vi "Reorder Connector Pane Object Refs.vi"(8 "Error In":errorcluster, 10 "Connector Pane Patter":u32, 11 "Connector Pane Object Refs":refnum<vi>[](array[refnum])) -> (0 "Error Out":errorcluster, 3 "Connector Pane Object Refs":refnum<vi>[][](array[refnum]))   [LabVIEW 2011, in "LVH-Toolbox.lvlib" / "LVH-Front-Panel-Clean-Up.lvlib"]
uses:
  <vilib>/LabVIEW Hacker/LVH-Toolbox/Front Panel Clean Up/LVH-Front-Panel-Clean-Up.lvlib
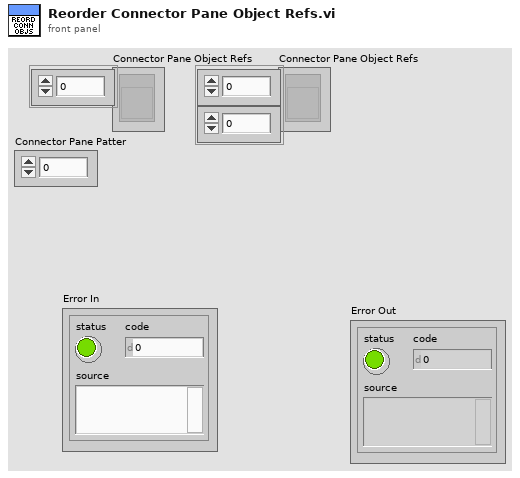
[diagram p1: front panel]
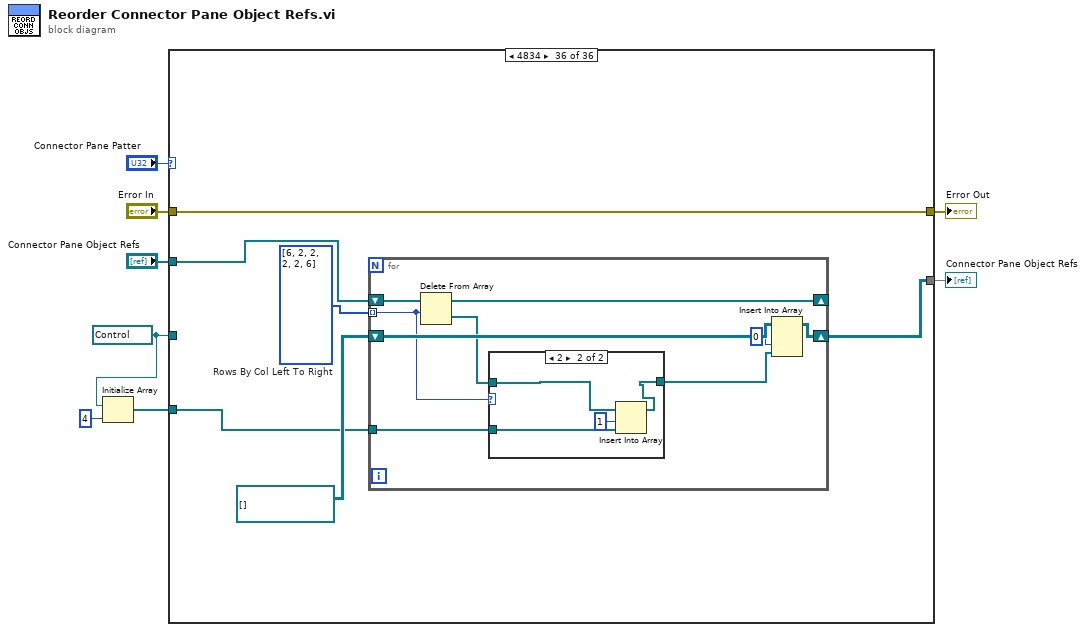
[diagram p0: block diagram]
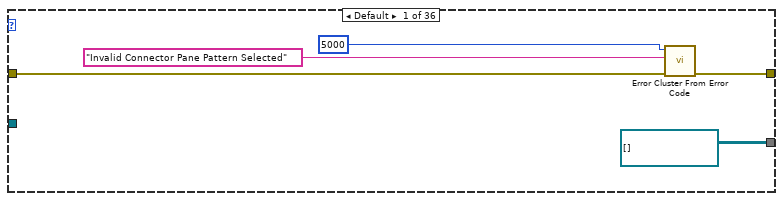
[diagram p2: hidden frame]
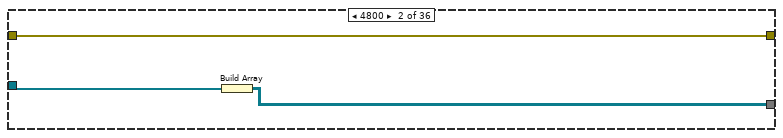
[diagram p3: hidden frame]
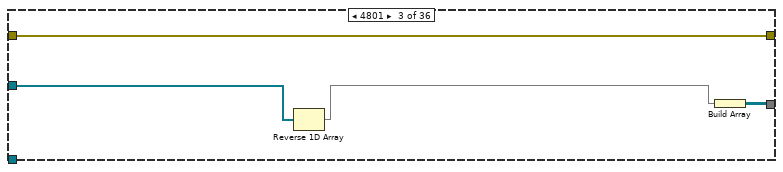
[diagram p4: hidden frame]
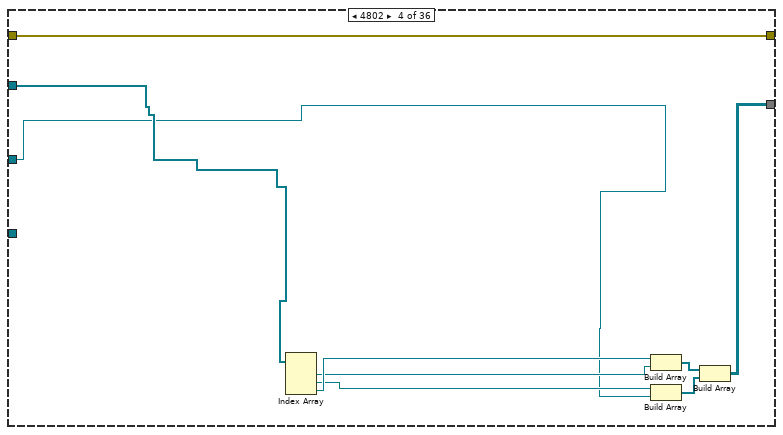
[diagram p5: hidden frame]
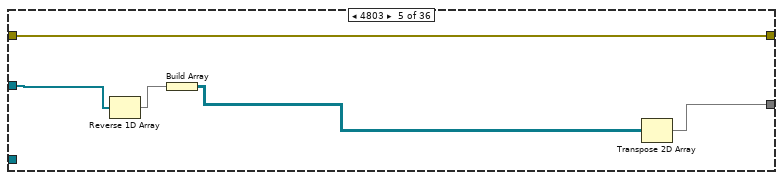
[diagram p6: hidden frame]
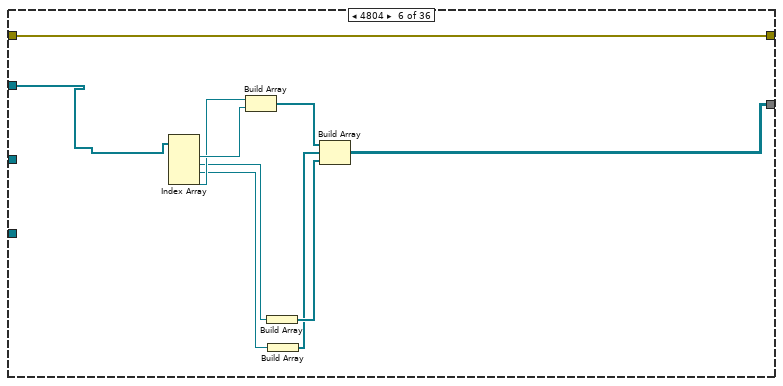
[diagram p7: hidden frame]
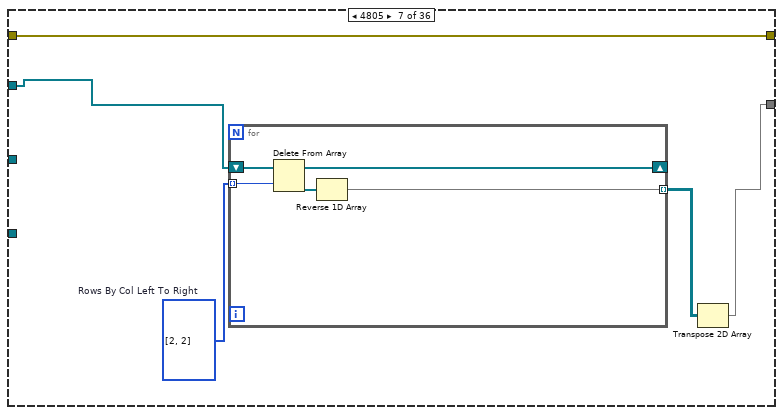
[diagram p8: hidden frame]
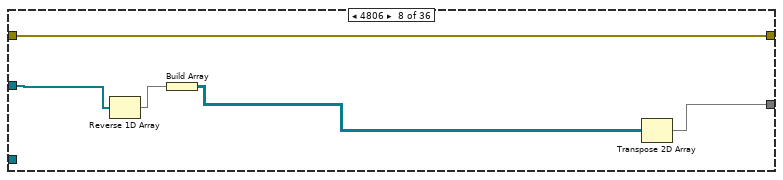
[diagram p9: hidden frame]
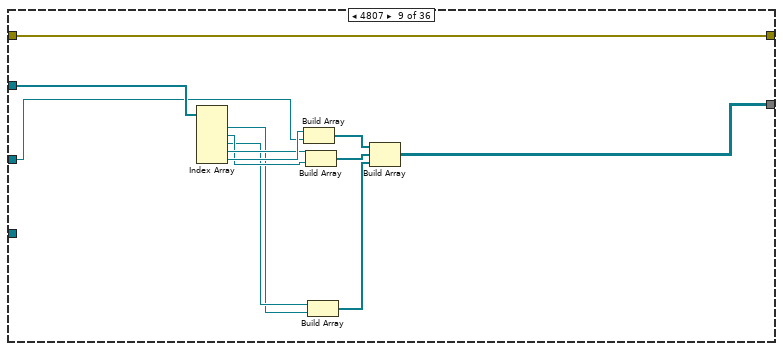
[diagram p10: hidden frame]
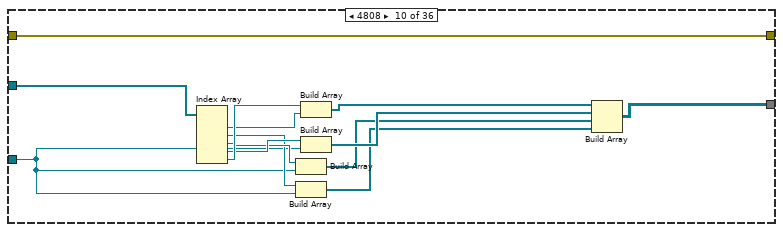
[diagram p11: hidden frame]
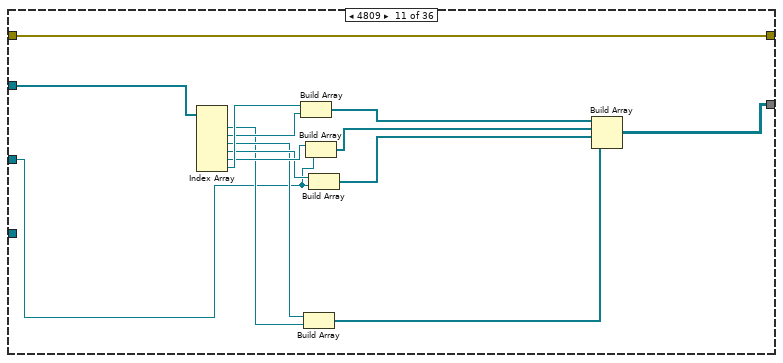
[diagram p12: hidden frame]
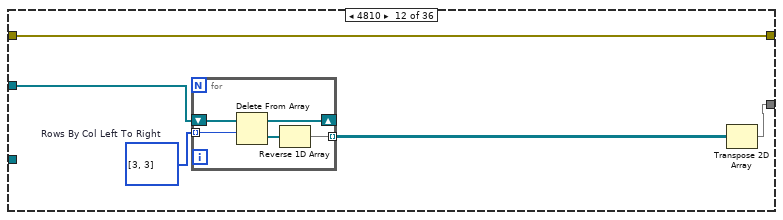
[diagram p13: hidden frame]
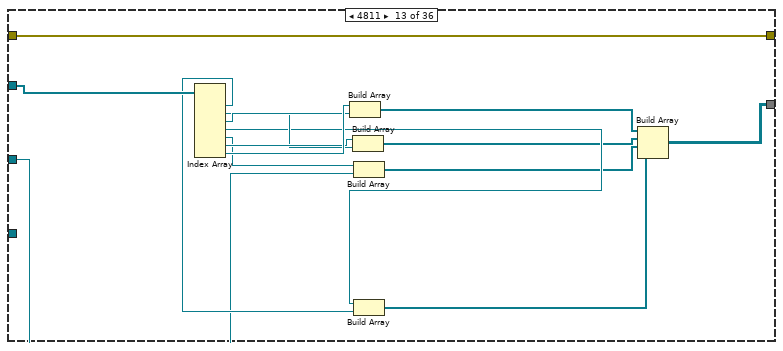
[diagram p14: hidden frame]
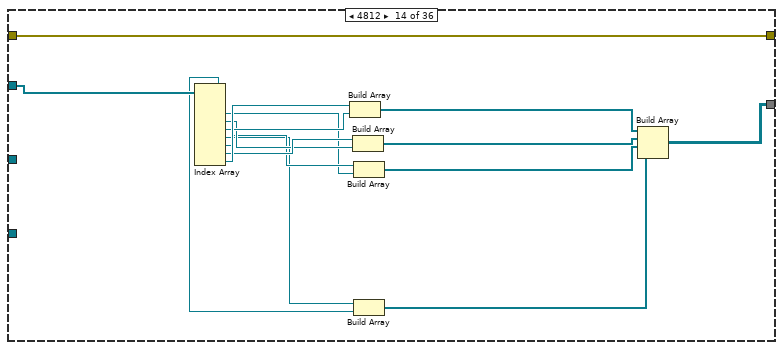
[diagram p15: hidden frame]
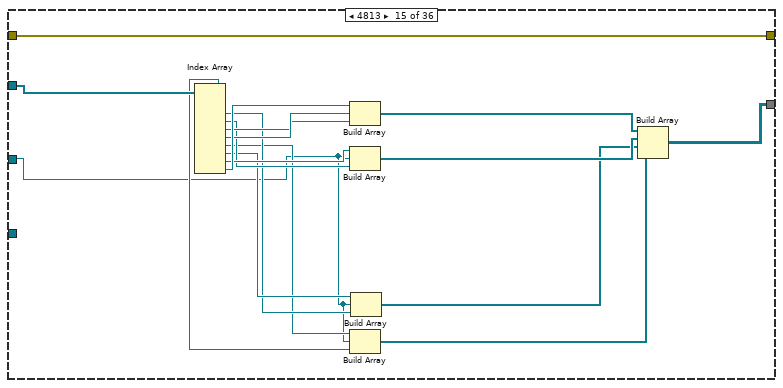
[diagram p16: hidden frame]
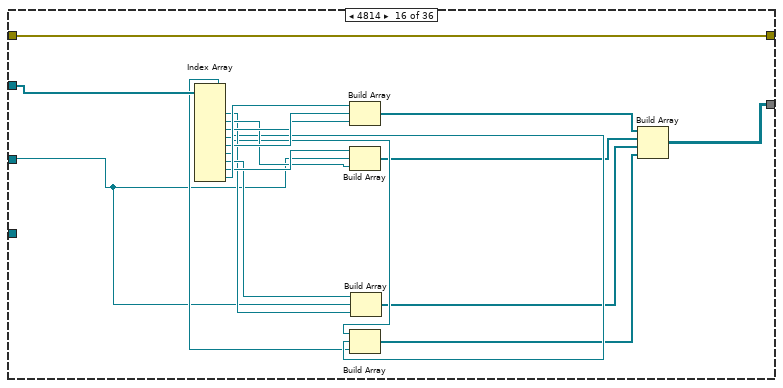
[diagram p17: hidden frame]
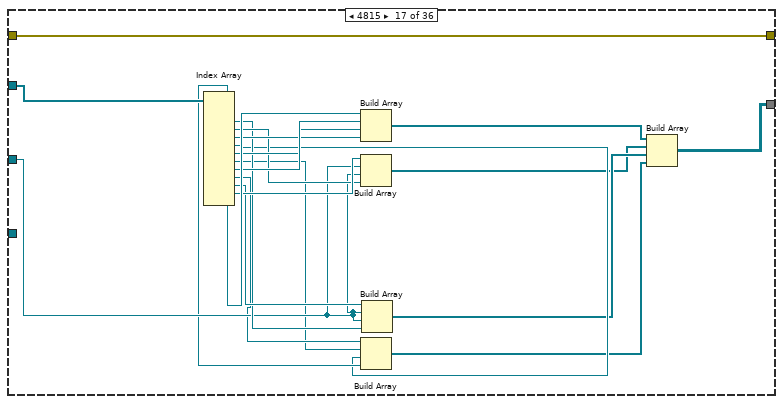
[diagram p18: hidden frame]
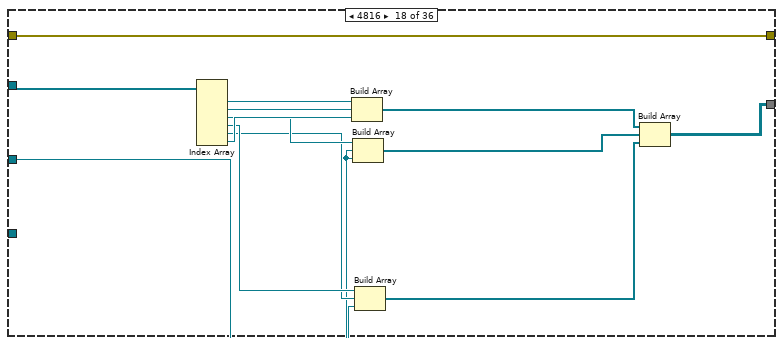
[diagram p19: hidden frame]
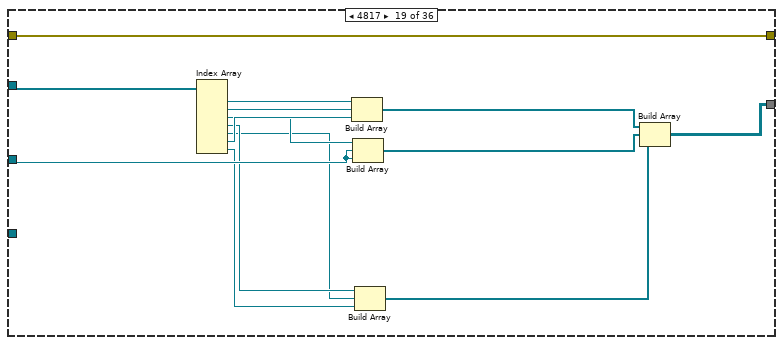
[diagram p20: hidden frame]
diagram:
  w2 = refnum<vi> refnum ("element")
  n1 = Initialize Array(w2, 4 ("dimension size")) -> (w1:refnum<vi>[])
  n2 = case shown="4834" "Connector Pane Patter" {
    tunnel: [w13 w14 w20 w29 w34 w44 w49 w59 w71 w84 w98 w103 w123 w138 w155 w173 w193 w206 w220 w235 w252 w269 w288 w305 w319 w334 w350 w368 w383 w399 w418 w428 w440 w453 w478 w484] -> w8
    tunnel: "Error In" -> [w10 w14 w20 w29 w34 w44 w49 w59 w71 w84 w98 w103 w123 w138 w155 w173 w193 w206 w220 w235 w252 w269 w288 w305 w319 w334 w350 w368 w383 w399 w418 w428 w440 w453 w478 w484]
    tunnel: "Connector Pane Object Refs" -> [_ w16 w18 w28 w31 w43 w47 w56 w70 w83 w97 w100 w122 w137 w154 w172 w192 w205 w219 w234 w251 w268 w287 w304 w318 w333 w349 w367 w382 w398 w417 w427 w439 w452 w468 w483]
    tunnel: [refnum<vi>[][] [] ("Connector Pane Object Refs") w15 w19 w22 w32 w38 w46 w57 w61 w73 w86 w99 w110 w124 w139 w156 w174 w195 w207 w221 w236 w253 w270 w289 w306 w321 w335 w351 w371 w384 w400 w420 w430 w451 w465 w479] -> w5
    tunnel: w2 -> [_ _ _ w21 _ _ _ _ w60 w72 w85 _ w109 _ w144 w157 w183 w194 w214 w228 w244 w262 w279 w297 w307 w320 w340 w356 w369 w392 w405 w419 w429 w441 w454 _]
    tunnel: w1 -> [_ _ _ _ _ _ _ _ _ _ _ _ _ _ _ _ _ _ _ _ _ _ _ _ _ _ _ _ _ _ _ _ _ _ _ w480]
    frame Default {
      n3 = call <vilib>:"Error Cluster From Error Code.vi"("error in (no error)"=w10, "error message (\"\")"="Invalid Connector Pane Pattern Selected" ("error message (\"\")"), "error code (0)"=5000) -> ("error out"=w13:errorcluster)  [unwired: 6 in]
    }
    frame 4800 {
      n4 = Build Array(w16) -> (w15:refnum<vi>[][])
    }
    frame 4801 {
      n5 = Reverse 1D Array(array=w18) -> (reversed array=w17:refnum<vi>[])
      n6 = Build Array(w17) -> (w19:refnum<vi>[][])
    }
    frame 4802 {
      n7 = Index Array(array=w28) -> (element #1=w26:refnum<vi>, element #2=w25:refnum<vi>, element #3=w27:refnum<vi>)  [unwired: 3 in]
      n8 = Build Array(w27, w26) -> (w24:refnum<vi>[])
      n9 = Build Array(w25, w21) -> (w23:refnum<vi>[])
      n10 = Build Array(w24, w23) -> (w22:refnum<vi>[][])
    }
    frame 4803 {
      n11 = Reverse 1D Array(array=w31) -> (reversed array=w30:refnum<vi>[])
      n12 = Build Array(w30) -> (w33:refnum<vi>[][])
      n13 = Transpose 2D Array(2D array=w33) -> (transposed array=w32:refnum<vi>[][])
    }
    frame 4804 {
      n14 = Index Array(array=w43) -> (element #1=w42:refnum<vi>, element #2=w40:refnum<vi>, element #3=w37:refnum<vi>, element #4=w41:refnum<vi>)  [unwired: 4 in]
      n15 = Build Array(w41, w42) -> (w39:refnum<vi>[])
      n16 = Build Array(w40) -> (w36:refnum<vi>[])
      n17 = Build Array(w37) -> (w35:refnum<vi>[])
      n18 = Build Array(w39, w35, w36) -> (w38:refnum<vi>[][])
    }
    frame 4805 {
      w48 = i32[] [2, 2]  # Rows By Col Left To Right
      n19 = for {
        tunnel: [w53] -> w45 mode=indexing
        shift-right: [w54] -> _
        shift-left: w47 -> [w52]
        tunnel: w48 -> [w50] mode=indexing
        n20 = Delete From Array(array=w52, length=w50) -> (deleted portion=w51:refnum<vi>[], array with subset deleted=w54:refnum<vi>[])  [unwired: 1 in]
        n21 = Reverse 1D Array(array=w51) -> (reversed array=w53:refnum<vi>[])
      }
      n22 = Transpose 2D Array(2D array=w45) -> (transposed array=w46:refnum<vi>[][])
    }
    frame 4806 {
      n23 = Reverse 1D Array(array=w56) -> (reversed array=w55:refnum<vi>[])
      n24 = Build Array(w55) -> (w58:refnum<vi>[][])
      n25 = Transpose 2D Array(2D array=w58) -> (transposed array=w57:refnum<vi>[][])
    }
    frame 4807 {
      n26 = Index Array(array=w70) -> (element #1=w65:refnum<vi>, element #2=w67:refnum<vi>, element #3=w66:refnum<vi>, element #4=w68:refnum<vi>, element #5=w69:refnum<vi>)  [unwired: 5 in]
      n27 = Build Array(w69, w60) -> (w64:refnum<vi>[])
      n28 = Build Array(w68, w67) -> (w63:refnum<vi>[])
      n29 = Build Array(w66, w65) -> (w62:refnum<vi>[])
      n30 = Build Array(w64, w63, w62) -> (w61:refnum<vi>[][])
    }
    frame 4808 {
      n31 = Index Array(array=w83) -> (element #1=w81:refnum<vi>, element #2=w78:refnum<vi>, element #3=w79:refnum<vi>, element #4=w80:refnum<vi>, element #5=w82:refnum<vi>)  [unwired: 5 in]
      n32 = Build Array(w79, w72) -> (w75:refnum<vi>[])
      n33 = Build Array(w78, w72) -> (w74:refnum<vi>[])
      n34 = Build Array(w82, w81) -> (w77:refnum<vi>[])
      n35 = Build Array(w80, w72) -> (w76:refnum<vi>[])
      n36 = Build Array(w77, w76, w75, w74) -> (w73:refnum<vi>[][])
    }
    frame 4809 {
      n37 = Index Array(array=w97) -> (element #1=w91:refnum<vi>, element #2=w95:refnum<vi>, element #3=w92:refnum<vi>, element #4=w93:refnum<vi>, element #5=w94:refnum<vi>, element #6=w96:refnum<vi>)  [unwired: 6 in]
      n38 = Build Array(w96, w95) -> (w90:refnum<vi>[])
      n39 = Build Array(w92, w91) -> (w87:refnum<vi>[])
      n40 = Build Array(w94, w85) -> (w89:refnum<vi>[])
      n41 = Build Array(w93, w85) -> (w88:refnum<vi>[])
      n42 = Build Array(w90, w89, w88, w87) -> (w86:refnum<vi>[][])
    }
    frame 4810 {
      w101 = i32[] [3, 3]  # Rows By Col Left To Right
      n43 = for {
        tunnel: [w107] -> w102 mode=indexing
        shift-right: [w108] -> _
        shift-left: w100 -> [w106]
        tunnel: w101 -> [w104] mode=indexing
        n44 = Delete From Array(array=w106, length=w104) -> (deleted portion=w105:refnum<vi>[], array with subset deleted=w108:refnum<vi>[])  [unwired: 1 in]
        n45 = Reverse 1D Array(array=w105) -> (reversed array=w107:refnum<vi>[])
      }
      n46 = Transpose 2D Array(2D array=w102) -> (transposed array=w99:refnum<vi>[][])
    }
    frame 4811 {
      n47 = Index Array(array=w122) -> (element #1=w115:refnum<vi>, element #2=w118:refnum<vi>, element #3=w120:refnum<vi>, element #4=w116:refnum<vi>, element #5=w117:refnum<vi>, element #6=w119:refnum<vi>, element #7=w121:refnum<vi>)  [unwired: 7 in]
      n48 = Build Array(w121, w120) -> (w114:refnum<vi>[])
      n49 = Build Array(w119, w118) -> (w113:refnum<vi>[])
      n50 = Build Array(w117, w109) -> (w112:refnum<vi>[])
      n51 = Build Array(w116, w115) -> (w111:refnum<vi>[])
      n52 = Build Array(w114, w113, w112, w111) -> (w110:refnum<vi>[][])
    }
    frame 4812 {
      n53 = Index Array(array=w137) -> (element #1=w129:refnum<vi>, element #2=w131:refnum<vi>, element #3=w133:refnum<vi>, element #4=w135:refnum<vi>, element #5=w130:refnum<vi>, element #6=w132:refnum<vi>, element #7=w134:refnum<vi>, element #8=w136:refnum<vi>)  [unwired: 8 in]
      n54 = Build Array(w136, w135) -> (w128:refnum<vi>[])
      n55 = Build Array(w134, w133) -> (w127:refnum<vi>[])
      n56 = Build Array(w132, w131) -> (w126:refnum<vi>[])
      n57 = Build Array(w130, w129) -> (w125:refnum<vi>[])
      n58 = Build Array(w128, w127, w126, w125) -> (w124:refnum<vi>[][])
    }
    frame 4813 {
      n59 = Index Array(array=w154) -> (element #1=w145:refnum<vi>, element #2=w147:refnum<vi>, element #3=w149:refnum<vi>, element #4=w151:refnum<vi>, element #5=w152:refnum<vi>, element #6=w146:refnum<vi>, element #7=w148:refnum<vi>, element #8=w150:refnum<vi>, element #9=w153:refnum<vi>)  [unwired: 9 in]
      n60 = Build Array(w153, w152, w151) -> (w143:refnum<vi>[])
      n61 = Build Array(w150, w144, w149) -> (w142:refnum<vi>[])
      n62 = Build Array(w146, w144, w145) -> (w140:refnum<vi>[])
      n63 = Build Array(w148, w144, w147) -> (w141:refnum<vi>[])
      n64 = Build Array(w143, w142, w141, w140) -> (w139:refnum<vi>[][])
    }
    frame 4814 {
      n65 = Index Array(array=w172) -> (element #1=w162:refnum<vi>, element #2=w165:refnum<vi>, element #3=w167:refnum<vi>, element #4=w169:refnum<vi>, element #5=w163:refnum<vi>, element #6=w170:refnum<vi>, element #7=w164:refnum<vi>, element #8=w166:refnum<vi>, element #9=w168:refnum<vi>, element #10=w171:refnum<vi>)  [unwired: 10 in]
      n66 = Build Array(w171, w170, w169) -> (w158:refnum<vi>[])
      n67 = Build Array(w168, w157, w167) -> (w159:refnum<vi>[])
      n68 = Build Array(w164, w163, w162) -> (w161:refnum<vi>[])
      n69 = Build Array(w166, w157, w165) -> (w160:refnum<vi>[])
      n70 = Build Array(w158, w159, w160, w161) -> (w156:refnum<vi>[][])
    }
    frame 4815 {
      n71 = Index Array(array=w192) -> (element #1=w181:refnum<vi>, element #2=w184:refnum<vi>, element #3=w186:refnum<vi>, element #4=w188:refnum<vi>, element #5=w179:refnum<vi>, element #6=w189:refnum<vi>, element #7=w180:refnum<vi>, element #8=w190:refnum<vi>, element #9=w182:refnum<vi>, element #10=w185:refnum<vi>, element #11=w187:refnum<vi>, element #12=w191:refnum<vi>)  [unwired: 12 in]
      n72 = Build Array(w191, w190, w189, w188) -> (w175:refnum<vi>[])
      n73 = Build Array(w187, w183, w183, w186) -> (w176:refnum<vi>[])
      n74 = Build Array(w182, w180, w179, w181) -> (w178:refnum<vi>[])
      n75 = Build Array(w185, w183, w183, w184) -> (w177:refnum<vi>[])
      n76 = Build Array(w175, w176, w177, w178) -> (w174:refnum<vi>[][])
    }
    frame 4816 {
      n77 = Index Array(array=w205) -> (element #1=w204:refnum<vi>, element #2=w203:refnum<vi>, element #3=w201:refnum<vi>, element #4=w200:refnum<vi>, element #5=w199:refnum<vi>, element #6=w202:refnum<vi>)  [unwired: 6 in]
      n78 = Build Array(w204, w203, w202) -> (w198:refnum<vi>[])
      n79 = Build Array(w201, w194, w194) -> (w197:refnum<vi>[])
      n80 = Build Array(w200, w199, w194) -> (w196:refnum<vi>[])
      n81 = Build Array(w198, w197, w196) -> (w195:refnum<vi>[][])
    }
    frame 4817 {
      n82 = Index Array(array=w219) -> (element #1=w218:refnum<vi>, element #2=w217:refnum<vi>, element #3=w215:refnum<vi>, element #4=w213:refnum<vi>, element #5=w212:refnum<vi>, element #6=w216:refnum<vi>, element #7=w211:refnum<vi>)  [unwired: 7 in]
      n83 = Build Array(w218, w217, w216) -> (w210:refnum<vi>[])
      n84 = Build Array(w215, w214, w214) -> (w209:refnum<vi>[])
      n85 = Build Array(w213, w212, w211) -> (w208:refnum<vi>[])
      n86 = Build Array(w210, w209, w208) -> (w207:refnum<vi>[][])
    }
    frame 4818 {
      n87 = Index Array(array=w234) -> (element #1=w233:refnum<vi>, element #2=w232:refnum<vi>, element #3=w230:refnum<vi>, element #4=w227:refnum<vi>, element #5=w226:refnum<vi>, element #6=w231:refnum<vi>, element #7=w229:refnum<vi>, element #8=w225:refnum<vi>)  [unwired: 8 in]
      n88 = Build Array(w233, w232, w231) -> (w224:refnum<vi>[])
      n89 = Build Array(w230, w228, w229) -> (w223:refnum<vi>[])
      n90 = Build Array(w227, w226, w225) -> (w222:refnum<vi>[])
      n91 = Build Array(w224, w223, w222) -> (w221:refnum<vi>[][])
    }
    frame 4819 {
      n92 = Index Array(array=w251) -> (element #1=w250:refnum<vi>, element #2=w249:refnum<vi>, element #3=w246:refnum<vi>, element #4=w243:refnum<vi>, element #5=w242:refnum<vi>, element #6=w248:refnum<vi>, element #7=w247:refnum<vi>, element #8=w245:refnum<vi>, element #9=w241:refnum<vi>)  [unwired: 9 in]
      n93 = Build Array(w250, w249, w248) -> (w240:refnum<vi>[])
      n94 = Build Array(w246, w244, w247) -> (w239:refnum<vi>[])
      n95 = Build Array(w243, w242, w241) -> (w237:refnum<vi>[])
      n96 = Build Array(w244, w244, w245) -> (w238:refnum<vi>[])
      n97 = Build Array(w240, w239, w238, w237) -> (w236:refnum<vi>[][])
    }
    frame 4820 {
      n98 = Index Array(array=w268) -> (element #1=w267:refnum<vi>, element #2=w266:refnum<vi>, element #3=w263:refnum<vi>, element #4=w260:refnum<vi>, element #5=w259:refnum<vi>, element #6=w265:refnum<vi>, element #7=w264:refnum<vi>, element #8=w261:refnum<vi>, element #9=w258:refnum<vi>, element #10=w257:refnum<vi>)  [unwired: 10 in]
      n99 = Build Array(w267, w266, w265, w264) -> (w256:refnum<vi>[])
      n100 = Build Array(w263, w262, w262, w261) -> (w255:refnum<vi>[])
      n101 = Build Array(w260, w259, w258, w257) -> (w254:refnum<vi>[])
      n102 = Build Array(w256, w255, w254) -> (w253:refnum<vi>[][])
    }
    frame 4821 {
      n103 = Index Array(array=w287) -> (element #1=w286:refnum<vi>, element #2=w285:refnum<vi>, element #3=w282:refnum<vi>, element #4=w278:refnum<vi>, element #5=w277:refnum<vi>, element #6=w284:refnum<vi>, element #7=w283:refnum<vi>, element #8=w281:refnum<vi>, element #9=w275:refnum<vi>, element #10=w280:refnum<vi>, element #11=w276:refnum<vi>)  [unwired: 11 in]
      n104 = Build Array(w286, w285, w284, w283) -> (w274:refnum<vi>[])
      n105 = Build Array(w282, w279, w279, w281) -> (w273:refnum<vi>[])
      n106 = Build Array(w279, w279, w279, w280) -> (w272:refnum<vi>[])
      n107 = Build Array(w278, w277, w275, w276) -> (w271:refnum<vi>[])
      n108 = Build Array(w274, w273, w272, w271) -> (w270:refnum<vi>[][])
    }
    frame 4822 {
      n109 = Index Array(array=w304) -> (element #1=w303:refnum<vi>, element #2=w302:refnum<vi>, element #3=w300:refnum<vi>, element #4=w298:refnum<vi>, element #5=w295:refnum<vi>, element #6=w296:refnum<vi>, element #7=w301:refnum<vi>, element #8=w299:refnum<vi>, element #9=w294:refnum<vi>)  [unwired: 9 in]
      n110 = Build Array(w303, w302, w301) -> (w293:refnum<vi>[])
      n111 = Build Array(w300, w297, w299) -> (w292:refnum<vi>[])
      n112 = Build Array(w298, w297, w297) -> (w291:refnum<vi>[])
      n113 = Build Array(w296, w295, w294) -> (w290:refnum<vi>[])
      n114 = Build Array(w293, w292, w291, w290) -> (w289:refnum<vi>[][])
    }
    frame 4823 {
      n115 = Index Array(array=w318) -> (element #1=w317:refnum<vi>, element #2=w314:refnum<vi>, element #3=w313:refnum<vi>, element #4=w312:refnum<vi>, element #5=w316:refnum<vi>, element #6=w315:refnum<vi>)  [unwired: 6 in]
      n116 = Build Array(w317, w316, w315) -> (w311:refnum<vi>[])
      n117 = Build Array(w314, w307, w307) -> (w310:refnum<vi>[])
      n118 = Build Array(w313, w307, w307) -> (w309:refnum<vi>[])
      n119 = Build Array(w312, w307, w307) -> (w308:refnum<vi>[])
      n120 = Build Array(w311, w310, w309, w308) -> (w306:refnum<vi>[][])
    }
    frame 4824 {
      n121 = Index Array(array=w333) -> (element #1=w332:refnum<vi>, element #2=w329:refnum<vi>, element #3=w328:refnum<vi>, element #4=w327:refnum<vi>, element #5=w331:refnum<vi>, element #6=w330:refnum<vi>, element #7=w326:refnum<vi>)  [unwired: 7 in]
      n122 = Build Array(w332, w331, w330) -> (w325:refnum<vi>[])
      n123 = Build Array(w329, w320, w320) -> (w324:refnum<vi>[])
      n124 = Build Array(w328, w320, w320) -> (w323:refnum<vi>[])
      n125 = Build Array(w327, w320, w326) -> (w322:refnum<vi>[])
      n126 = Build Array(w325, w324, w323, w322) -> (w321:refnum<vi>[][])
    }
    frame 4825 {
      n127 = Index Array(array=w349) -> (element #1=w348:refnum<vi>, element #2=w345:refnum<vi>, element #3=w343:refnum<vi>, element #4=w342:refnum<vi>, element #5=w347:refnum<vi>, element #6=w346:refnum<vi>, element #7=w344:refnum<vi>, element #8=w341:refnum<vi>)  [unwired: 8 in]
      n128 = Build Array(w348, w347, w346) -> (w339:refnum<vi>[])
      n129 = Build Array(w345, w340, w344) -> (w338:refnum<vi>[])
      n130 = Build Array(w343, w340, w340) -> (w337:refnum<vi>[])
      n131 = Build Array(w342, w340, w341) -> (w336:refnum<vi>[])
      n132 = Build Array(w339, w338, w337, w336) -> (w335:refnum<vi>[][])
    }
    frame 4826 {
      n133 = Index Array(array=w367) -> (element #1=w357:refnum<vi>, element #2=w358:refnum<vi>, element #3=w361:refnum<vi>, element #4=w363:refnum<vi>, element #5=w364:refnum<vi>, element #6=w365:refnum<vi>, element #7=w359:refnum<vi>, element #8=w360:refnum<vi>, element #9=w362:refnum<vi>, element #10=w366:refnum<vi>)  [unwired: 10 in]
      n134 = Build Array(w360, w356, w356, w358) -> (w353:refnum<vi>[])
      n135 = Build Array(w359, w356, w356, w357) -> (w352:refnum<vi>[])
      n136 = Build Array(w366, w365, w364, w363) -> (w355:refnum<vi>[])
      n137 = Build Array(w362, w356, w356, w361) -> (w354:refnum<vi>[])
      n138 = Build Array(w355, w354, w353, w352) -> (w351:refnum<vi>[][])
    }
    frame 4827 {
      n139 = Index Array(array=w382) -> (element #1=w379:refnum<vi>, element #2=w370:refnum<vi>, element #3=w380:refnum<vi>, element #4=w376:refnum<vi>, element #5=w377:refnum<vi>, element #6=w378:refnum<vi>, element #7=w381:refnum<vi>)  [unwired: 7 in]
      n140 = Build Array(w377, w369, w369) -> (w373:refnum<vi>[])
      n141 = Build Array(w376, w370, w369) -> (w372:refnum<vi>[])
      n142 = Build Array(w381, w380, w379) -> (w375:refnum<vi>[])
      n143 = Build Array(w378, w369, w369) -> (w374:refnum<vi>[])
      n144 = Build Array(w375, w374, w373, w372) -> (w371:refnum<vi>[][])
    }
    frame 4828 {
      n145 = Index Array(array=w398) -> (element #1=w389:refnum<vi>, element #2=w395:refnum<vi>, element #3=w390:refnum<vi>, element #4=w396:refnum<vi>, element #5=w391:refnum<vi>, element #6=w393:refnum<vi>, element #7=w394:refnum<vi>, element #8=w397:refnum<vi>)  [unwired: 8 in]
      n146 = Build Array(w393, w392, w392) -> (w386:refnum<vi>[])
      n147 = Build Array(w391, w390, w389) -> (w385:refnum<vi>[])
      n148 = Build Array(w397, w396, w395) -> (w388:refnum<vi>[])
      n149 = Build Array(w394, w392, w392) -> (w387:refnum<vi>[])
      n150 = Build Array(w388, w387, w386, w385) -> (w384:refnum<vi>[][])
    }
    frame 4829 {
      n151 = Index Array(array=w417) -> (element #1=w406:refnum<vi>, element #2=w409:refnum<vi>, element #3=w411:refnum<vi>, element #4=w414:refnum<vi>, element #5=w413:refnum<vi>, element #6=w407:refnum<vi>, element #7=w415:refnum<vi>, element #8=w408:refnum<vi>, element #9=w410:refnum<vi>, element #10=w412:refnum<vi>, element #11=w416:refnum<vi>)  [unwired: 11 in]
      n152 = Build Array(w408, w407, w405, w406) -> (w401:refnum<vi>[])
      n153 = Build Array(w410, w405, w405, w409) -> (w402:refnum<vi>[])
      n154 = Build Array(w416, w415, w413, w414) -> (w404:refnum<vi>[])
      n155 = Build Array(w412, w405, w405, w411) -> (w403:refnum<vi>[])
      n156 = Build Array(w404, w403, w402, w401) -> (w400:refnum<vi>[][])
    }
    frame 4830 {
      n157 = Index Array(array=w427) -> (element #1=w424:refnum<vi>, element #2=w425:refnum<vi>, element #3=w423:refnum<vi>, element #4=w426:refnum<vi>)  [unwired: 4 in]
      n158 = Build Array(w426, w425, w424) -> (w422:refnum<vi>[])
      n159 = Build Array(w423, w419, w419) -> (w421:refnum<vi>[])
      n160 = Build Array(w422, w421) -> (w420:refnum<vi>[][])
    }
    frame 4831 {
      n161 = Index Array(array=w439) -> (element #1=w435:refnum<vi>, element #2=w436:refnum<vi>, element #3=w434:refnum<vi>, element #4=w437:refnum<vi>, element #5=w438:refnum<vi>)  [unwired: 5 in]
      n162 = Build Array(w438, w436, w435) -> (w433:refnum<vi>[])
      n163 = Build Array(w437, w429, w429) -> (w432:refnum<vi>[])
      n164 = Build Array(w434, w429, w429) -> (w431:refnum<vi>[])
      n165 = Build Array(w433, w432, w431) -> (w430:refnum<vi>[][])
    }
    frame 4832 {
      n166 = Index Array(array=w452) -> (element #1=w445:refnum<vi>, element #2=w448:refnum<vi>, element #3=w449:refnum<vi>, element #4=w446:refnum<vi>, element #5=w447:refnum<vi>, element #6=w450:refnum<vi>)  [unwired: 6 in]
      n167 = Build Array(w450, w449, w448) -> (w444:refnum<vi>[])
      n168 = Build Array(w446, w441, w445) -> (w442:refnum<vi>[])
      n169 = Build Array(w447, w441, w441) -> (w443:refnum<vi>[])
      n170 = Build Array(w444, w443, w442) -> (w451:refnum<vi>[][])
    }
    frame 4833 {
      (unwired) 5 ("length")
      n171 = Array Subset(array=w468, index=11 ("length"), length=5) -> (w455:refnum<vi>[])
      n172 = Array Subset(array=w468, index=9 ("length"), length=2) -> (w459:refnum<vi>[])
      n173 = Array Subset(array=w468, index=7 ("length"), length=2) -> (w460:refnum<vi>[])
      n174 = Array Subset(array=w468, index=5 ("length"), length=2) -> (w464:refnum<vi>[])
      n175 = Array Subset(array=w468, index=0, length=5) -> (w466:refnum<vi>[])
      n176 = Insert Into Array(array=w464, index=1, new element #1=w454, new element #2=w454, new element #3=w454) -> (w458:refnum<vi>[])
      n177 = Insert Into Array(array=w460, index=1, new element #1=w454, new element #2=w454, new element #3=w454) -> (w457:refnum<vi>[])
      n178 = Insert Into Array(array=w459, index=1, new element #1=w454, new element #2=w454, new element #3=w454) -> (w456:refnum<vi>[])
      n179 = Build Array(w466, w458, w457, w456, w455) -> (w465:refnum<vi>[][])
    }
    frame 4834 {
      w482 = i32[] [6, 2, 2, 2, 2, 6]  # Rows By Col Left To Right
      n180 = for {
        shift-right: [w493] -> _
        shift-left: w483 -> [w492]
        tunnel: w482 -> [w488] mode=indexing
        shift-right: [w490] -> w479
        shift-left: refnum<vi>[][] [] ("array") -> [w491]
        tunnel: w480 -> [w485]
        n181 = Delete From Array(array=w492, length=w488) -> (deleted portion=w486:refnum<vi>[], array with subset deleted=w493:refnum<vi>[])  [unwired: 1 in]
        n182 = case shown="2" w488 {
          tunnel: [w494 w495] -> w487
          tunnel: w486 -> [w494 w496]
          tunnel: w485 -> [_ w498]
          frame 0, Default {
            # "No Spacers Needed"
          }
          frame 2 {
            n183 = Insert Into Array(array=w496, index=1, new element=w498) -> (w495:refnum<vi>[])
          }
        }
        n184 = Insert Into Array(array=w491, index (col)=0 ("index (row)"), new element=w487) -> (w490:refnum<vi>[][])  [unwired: 1 in]
      }
    }
  }
  "Error Out" <- w8
  "Connector Pane Object Refs" <- w5
